vi "re_obj_LuaVIEW Task State.vi"(0 "method":T6, 1 "mode {set mode}":T2, 7 "signal":T1, 11 "script index":i32, 12 "string in":string) -> (6 "task info {get task info}":T4 {"handle mask" format="%.0b"; "allow mask" format="%.0b"; "signal flags" format="%.0b"}, 8 "set/available/pending":bool, 10 "script info":T3, 14 "string out":string, 15 "wakeup occurrence":refnum<k4>)   [LabVIEW 2012]
doc: "Instantiated per task. Holds the state of a task and allows for asynchronous communication with a task. Must be called by reference. A reference can be obtained from the task list.\n\nThis VI is only marginally part of the API: those methods that are in common use by function VIs can be deemed safe for use provided that typedefs are used so as to be forward compatible with extension of the method enum or typedef clusters (only use unbundle/bundle by name, and so on)."
uses:
  typedefs/t_LuaVIEW Task State Methods.ctl
  typedefs/t_LuaVIEW Task Modes.ctl
  typedefs/clusters/LuaVIEW Task Info.ctl
  typedefs/t_LuaVIEW Reference.ctl
  typedefs/t_LuaVIEW Task Signals.ctl
  typedefs/clusters/LuaVIEW Script Info.ctl
  typedefs/t_LuaVIEW Prepared Script Infos Methods.ctl
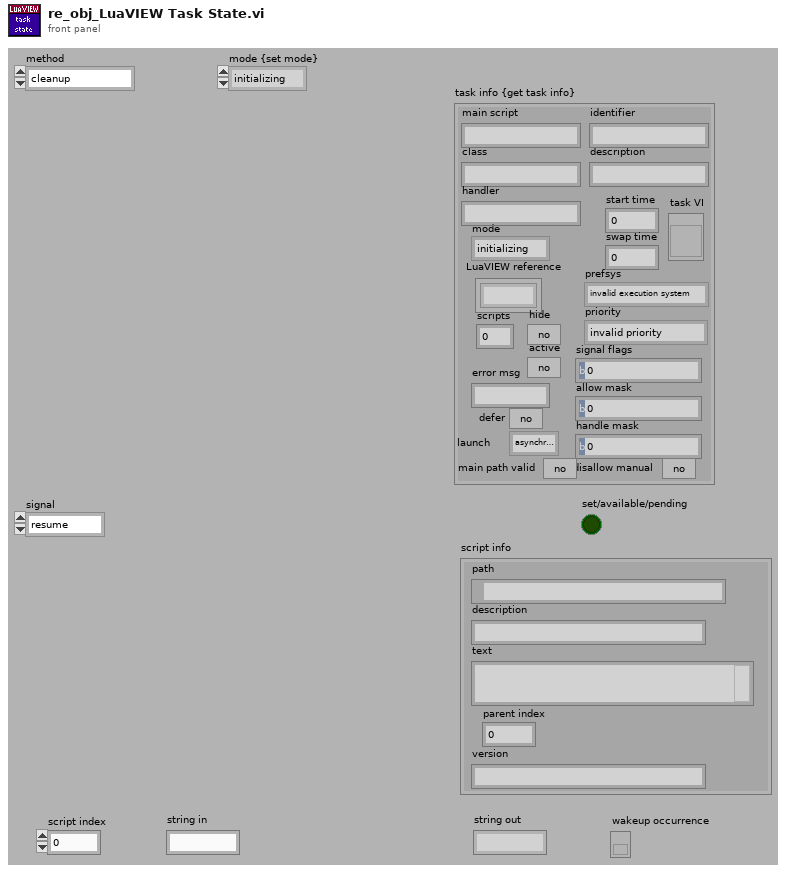
[diagram p1: front panel]
types:
  T1 = typedef "t_LuaVIEW Task Signals.ctl" = enum32{"resume", "pause", "swap", "stop", "confirm"}
  T2 = typedef "t_LuaVIEW Task Modes.ctl" = enum16{"initializing", "running", "executing", "paused", "error", "swapping"}
  T3 = typedef "LuaVIEW Script Info.ctl" = cluster{"path":path, "description":string, "text":string, "parent index":i32, "version":string}
  T4 = typedef "LuaVIEW Task Info.ctl" = cluster{"main script":string, "identifier":string, "class":string, "description":string, "mode":T2, "handler":string, "LuaVIEW reference":T5, "scripts":i32, "hide":bool, "active":bool, "error msg":string, "defer":bool, "launch":enum16{"asynchronous", "manual", "synchronous"}, "main path valid":bool, "start time":dbl, "swap time":dbl, "task VI":refnum<vi>, "prefsys":enum32{"invalid execution system", "user interface", "standard", "instrument i/o", "data acquisition", "other 1", "other 2", "same as caller"}, "priority":enum32{"invalid priority", "background priority", "normal priority", "above normal priority", "high priority", "time critical priority", "subroutine"}, "signal flags":u32, "allow mask":u32, "handle mask":u32, "disallow manual":bool}
  T5 = typedef "t_LuaVIEW Reference.ctl" = refnum<k1>
  T6 = typedef "t_LuaVIEW Task State Methods.ctl" = enum16{"cleanup", "set initial", "set mode", "set active mode", "set error", "get task info", "get script info", "set signal", "clear signal", "test handled", "test delegated", "test signal", "handle signal", "delegate signal", "allow signal", "disallow signal", "disallow all", "signals?", "delegated signals?", "protection++", "protection--", "protection=0", "message", "next message", "pop message", "message available?", "force stop", "set swap preps", "apply swap preps"}
  T7 = typedef "t_LuaVIEW Prepared Script Infos Methods.ctl" = enum16{"isempty?", "empty", "set", "discard"}
  T8 = enum32{"invalid execution system", "user interface", "standard", "instrument i/o", "data acquisition", "other 1", "other 2", "same as caller"}
  T9 = enum32{"invalid priority", "background priority", "normal priority", "above normal priority", "high priority", "time critical priority", "subroutine"}
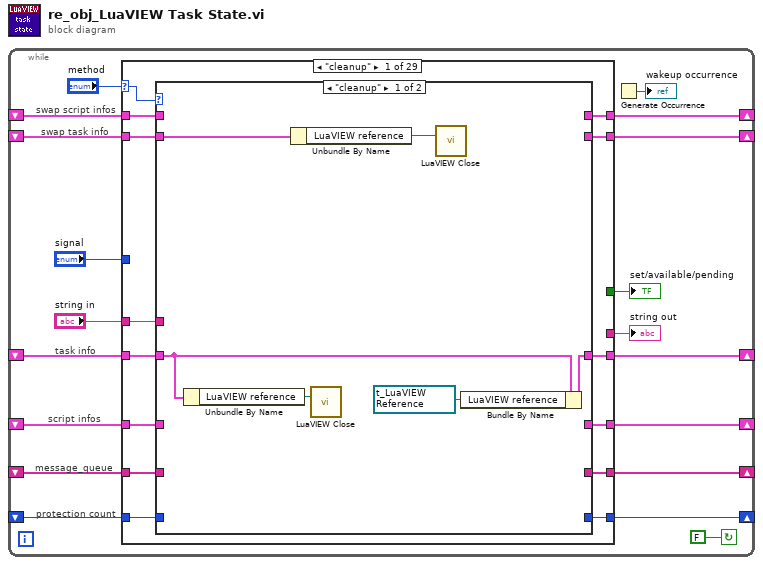
[diagram p0: block diagram]
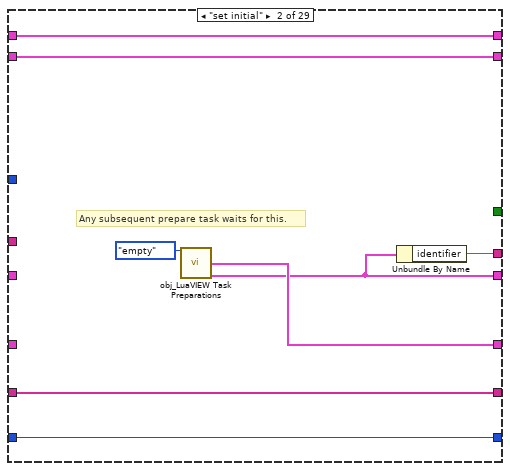
[diagram p3: hidden frame]
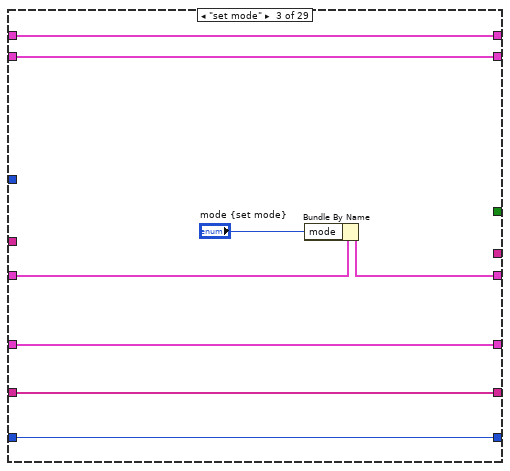
[diagram p4: hidden frame]
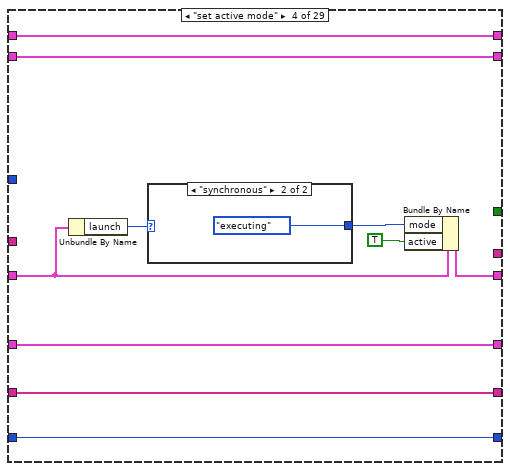
[diagram p5: hidden frame]
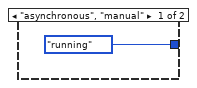
[diagram p6: hidden frame]
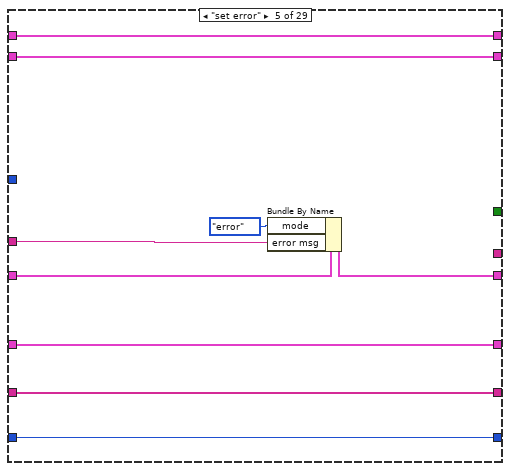
[diagram p7: hidden frame]
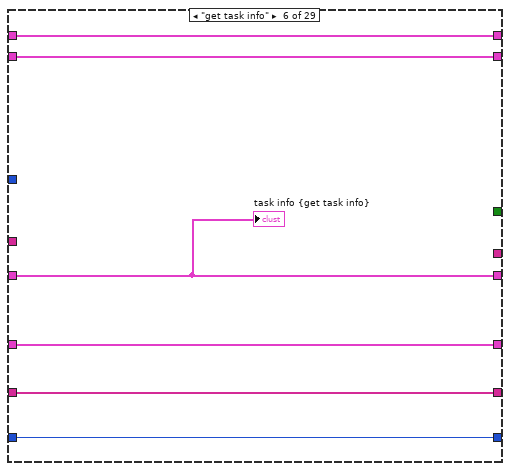
[diagram p8: hidden frame]
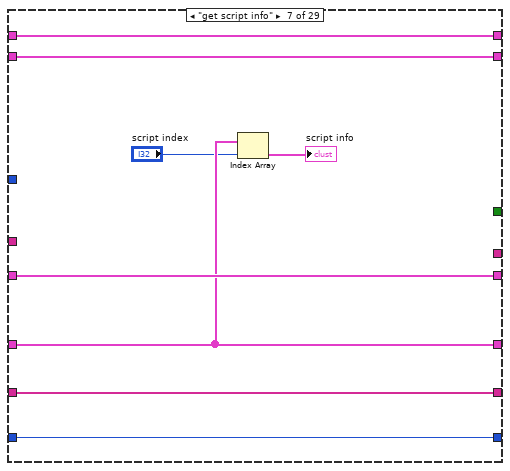
[diagram p9: hidden frame]
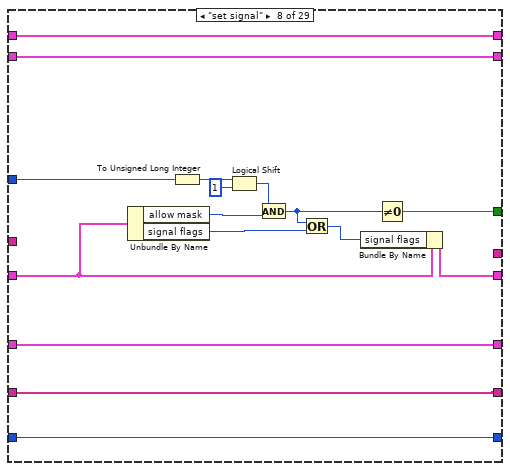
[diagram p10: hidden frame]
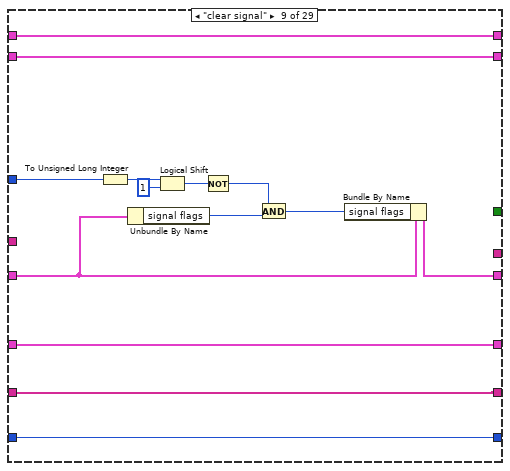
[diagram p11: hidden frame]
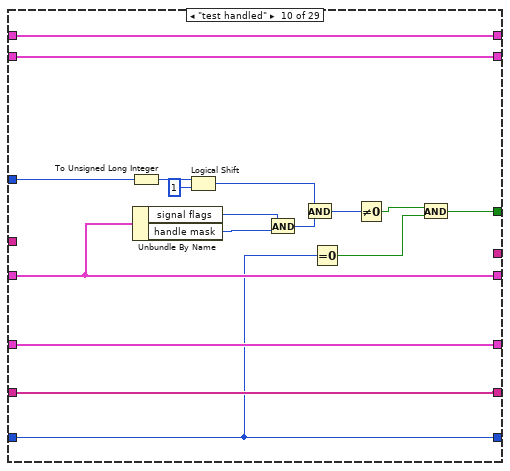
[diagram p12: hidden frame]
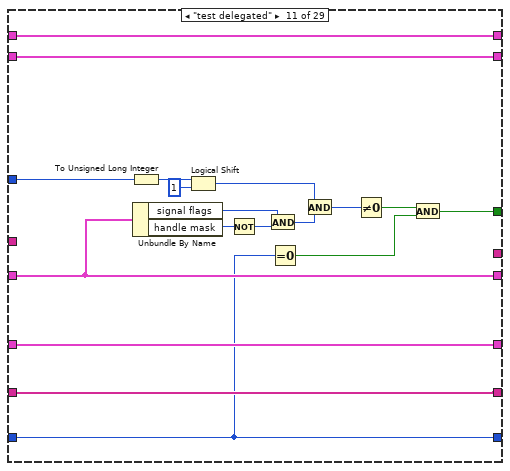
[diagram p13: hidden frame]
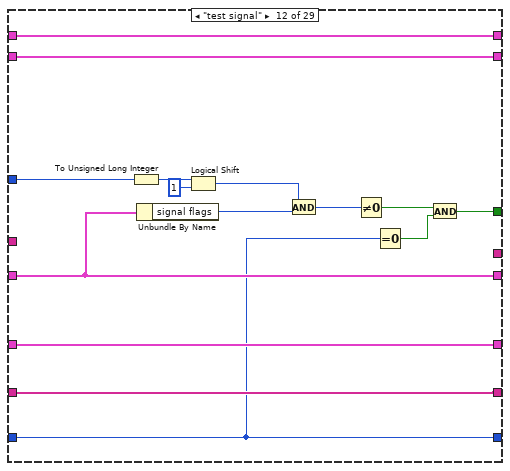
[diagram p14: hidden frame]
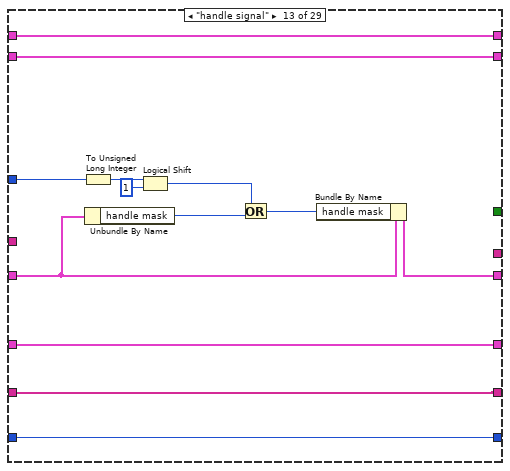
[diagram p15: hidden frame]
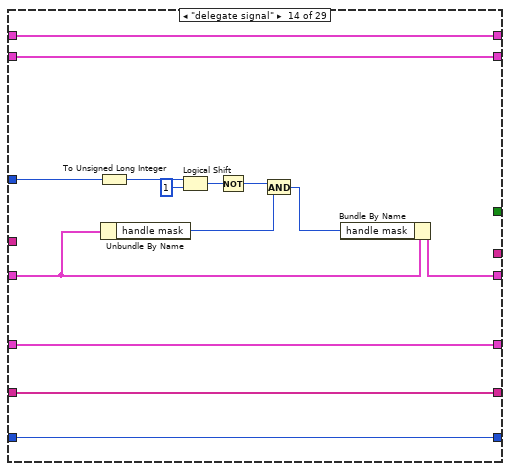
[diagram p16: hidden frame]
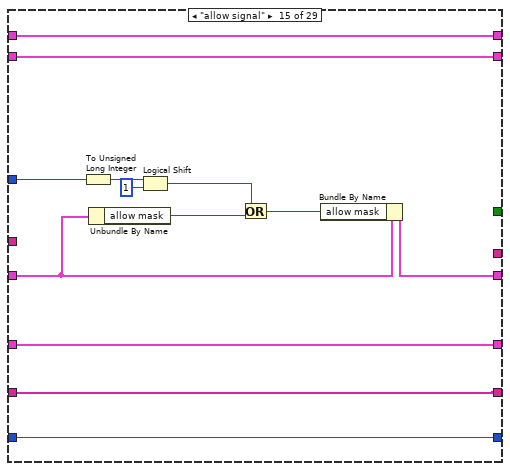
[diagram p17: hidden frame]
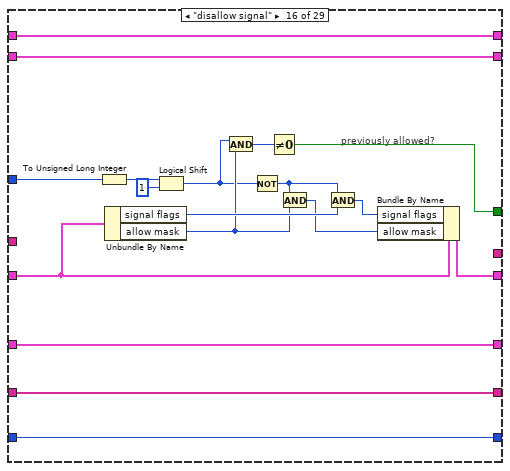
[diagram p18: hidden frame]
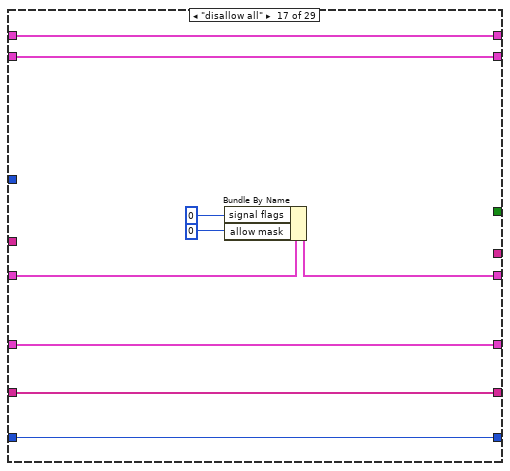
[diagram p19: hidden frame]
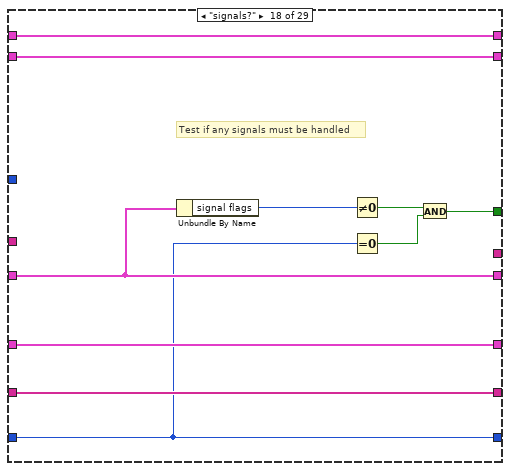
[diagram p20: hidden frame]
diagram:
  n1 = while {
    shift-right: [w17] -> _
    shift-left: _ -> [w16]
    shift-right: [w14] -> _
    shift-left: _ -> [w15]
    shift-right: [w9] -> _
    shift-left: _ -> [w10]
    shift-right: [w5] -> _
    shift-left: _ -> [w6]
    shift-right: [w1] -> _
    shift-left: _ -> [w4]
    shift-right: [w2] -> _
    shift-left: _ -> [w3]
    stop <- FALSE continue-if-true
    # "swap task info"
    # "swap script infos"
    # "protection count"
    # "message_queue"
    # "script infos"
    # "task info"
    n2 = case shown="\"cleanup\"" "method" {
      selector: "method" -> [w20 _ _ _ _ _ _ _ _ _ _ _ _ _ _ _ _ _ _ _ _ _ _ _ _ _ _ _ _]
      tunnel: [w31 w48 w59 w70 w82 w88 w96 w107 w121 w137 w155 w170 w182 w198 w209 w229 w241 w251 w264 w274 w284 w290 w298 w316 w334 w350 w364 w373 w412] -> w17
      tunnel: w16 -> [w33 _ w60 w67 w80 w88 w96 w108 w122 w137 w155 w170 w183 w199 w210 w230 w242 w251 w264 w274 w284 w290 w298 w316 w334 w350 w365 w374 w407]
      tunnel: w15 -> [w32 _ w61 w71 w81 w87 w95 w112 w126 w143 w161 w176 w189 w203 w216 w234 w243 w253 w266 w275 w285 w291 w302 w317 w335 w351 w368 w391 w413]
      tunnel: [w30 w50 w61 w71 w81 w87 w95 w112 w126 w143 w161 w176 w189 w203 w216 w234 w243 w253 w266 w275 w285 w291 w302 w317 w335 w351 w368 w391 w411] -> w14
      tunnel: "signal" -> [_ _ _ _ _ _ _ w109 w123 w138 w156 w171 w186 w200 w213 w231 _ _ _ _ _ _ _ _ _ _ _ _ _]
      tunnel: [_ _ _ _ _ _ _ w104 _ w132 w149 w167 _ _ _ w223 _ w249 w258 w270 w278 _ w295 w310 w328 w348 TRUE w376 w408] -> w12
      tunnel: w10 -> [w29 w53 w57 w69 w78 w86 w93 w100 w118 w136 w154 w168 w180 w195 w207 w222 w238 w250 w263 w273 w283 w289 w301 w313 w331 w347 w361 w384 w418]
      tunnel: [w28 w53 w57 w69 w78 w86 w93 w100 w118 w136 w154 w168 w180 w195 w207 w222 w238 w250 w263 w273 w283 w289 w300 w315 w333 w347 w361 w384 w418] -> w9
      tunnel: [_ w49 _ _ _ _ _ _ _ _ _ _ _ _ _ _ _ _ _ _ _ _ _ w314 w332 _ _ _ _] -> w8
      tunnel: "string in" -> [w27 _ _ _ w77 _ _ _ _ _ _ _ _ _ _ _ _ _ _ _ _ _ w299 _ _ _ _ _ _]
      tunnel: w6 -> [w21 w52 w56 w68 w76 w85 w92 w99 w117 w130 w147 w164 w179 w192 w206 w219 w237 w247 w256 w272 w282 _ w294 w309 w327 w346 w360 w383 _]
      tunnel: [w26 w52 w56 w68 w76 w85 w92 w99 w117 w130 w147 w164 w179 w192 w206 w219 w237 w247 w256 w271 w280 0 ("t") w294 w309 w327 w346 w360 w383 0 ("t")] -> w5
      tunnel: w4 -> [w25 w47 w55 w64 w75 w84 w91 w98 w114 w128 w145 w163 w178 w191 w205 w218 w236 w246 w255 w268 w277 w287 w293 w308 w326 w345 w353 w378 w410]
      tunnel: w3 -> [w24 w46 w54 w63 w74 w83 w90 w97 w113 w127 w144 w162 w177 w190 w204 w217 w235 w245 w254 w267 w276 w286 w292 w307 w325 w344 w352 w377 w417]
      tunnel: [w22 w46 w54 w63 w74 w83 w90 w97 w113 w127 w144 w162 w177 w190 w204 w217 w235 w245 w254 w267 w276 w286 w292 w307 w325 w344 w352 w380 w415] -> w2
      tunnel: [w23 w47 w55 w64 w75 w84 w91 w98 w114 w128 w145 w163 w178 w191 w205 w218 w236 w246 w255 w268 w277 w287 w293 w308 w326 w345 w353 w381 w416] -> w1
      frame "cleanup" {
        n3 = case shown="\"cleanup\"" w20 {
          tunnel: w33 -> [w37 w43]
          tunnel: w32 -> [_ w42]
          tunnel: [w36 w43] -> w31
          tunnel: [_ w42] -> w30
          tunnel: w29 -> [_ w41]
          tunnel: [_ w41] -> w28
          tunnel: w27 -> [_ _]
          tunnel: [_ w40] -> w26
          tunnel: w25 -> [_ w45]
          tunnel: w24 -> [w35 w44]
          tunnel: [_ w45] -> w23
          tunnel: [_ w44] -> w22
          tunnel: w21 -> [_ w40]
          frame "cleanup" {
            w34 = T5 refnum items=["LuaVIEW"] ("LuaVIEW reference")
            n4 = Unbundle By Name(w37) -> ("LuaVIEW reference"=w39:T5)
            n5 = Unbundle By Name(w35) -> ("LuaVIEW reference"=w38:T5)
            n6 = call "LuaVIEW Close.vi"("LuaVIEW reference"=w39) -> ()  [unwired: 14 in, 1 out]
            n7 = call "LuaVIEW Close.vi"("LuaVIEW reference"=w38) -> ()  [unwired: 14 in, 1 out]
            n8 = Bundle By Name(cluster=w37, "LuaVIEW reference"=w34) -> (w36:T4)
          }
          frame Default {
          }
        }
      }
      frame "set initial" {
        # "Any subsequent prepare task waits for this."
        n9 = call "obj_LuaVIEW Task Preparations.vi"("method"=t_LuaVIEW_Prepared_Script_Infos_Methods."empty") -> ("script infos out"=w50:T3[], "task info out"=w48:T4)  [unwired: 12 in, 1 out]
        n10 = Unbundle By Name(w48) -> ("identifier"=w49:string)
      }
      frame "set mode" {
        n11 = Bundle By Name(cluster=w60, "mode"="mode {set mode}") -> (w59:T4)
      }
      frame "set active mode" {
        n12 = Unbundle By Name(w67) -> ("launch"=w66:enum16{"asynchronous", "manual", "synchronous"})
        n13 = case shown="\"synchronous\"" w66 {
          tunnel: [t_LuaVIEW_Task_Modes."running" ("mode") t_LuaVIEW_Task_Modes."executing" ("mode")] -> w65
          frame "asynchronous", "manual" {
          }
          frame "synchronous" {
          }
        }
        n14 = Bundle By Name(cluster=w67, "mode"=w65, "active"=TRUE) -> (w70:T4)
      }
      frame "set error" {
        n15 = Bundle By Name(cluster=w80, "mode"=t_LuaVIEW_Task_Modes."error", "error msg"=w77) -> (w82:T4)
      }
      frame "get task info" {
        "task info {get task info}" <- w88
      }
      frame "get script info" {
        n16 = Index Array(array=w95, index="script index") -> (element=→"script info":T3)
      }
      frame "set signal" {
        n17 = Unbundle By Name(w108) -> ("allow mask"=w105:u32, "signal flags"=w103:u32)
        n18 = To Unsigned Long Integer(number=w109) -> (unsigned 32bit integer=w110:u32)
        n19 = Logical Shift(y=w110, x=u32 1) -> (x << y=w106:u32)
        n20 = And(x=w106, y=w105) -> (x .and. y?=w102:u32)
        n21 = Or(x=w102, y=w103) -> (x .or. y?=w101:u32)
        n22 = Bundle By Name(cluster=w108, "signal flags"=w101) -> (w107:T4)
        n23 = Not Equal To 0?(x=w102) -> (x != 0?=w104:bool)
      }
      frame "clear signal" {
        n24 = To Unsigned Long Integer(number=w123) -> (unsigned 32bit integer=w124:u32)
        n25 = Unbundle By Name(w122) -> ("signal flags"=w119:u32)
        n26 = Logical Shift(y=w124, x=u32 1) -> (x << y=w120:u32)
        n27 = Not(x=w120) -> (.not. x?=w115:u32)
        n28 = And(x=w115, y=w119) -> (x .and. y?=w116:u32)
        n29 = Bundle By Name(cluster=w122, "signal flags"=w116) -> (w121:T4)
      }
      frame "test handled" {
        n30 = To Unsigned Long Integer(number=w138) -> (unsigned 32bit integer=w141:u32)
        n31 = Unbundle By Name(w137) -> ("signal flags"=w135:u32, "handle mask"=w133:u32)
        n32 = Logical Shift(y=w141, x=u32 1) -> (x << y=w140:u32)
        n33 = And(x=w135, y=w133) -> (x .and. y?=w134:u32)
        n34 = And(x=w140, y=w134) -> (x .and. y?=w139:u32)
        n35 = Equal To 0?(x=w130) -> (x = 0?=w129:bool)
        n36 = Not Equal To 0?(x=w139) -> (x != 0?=w131:bool)
        n37 = And(x=w131, y=w129) -> (x .and. y?=w132:bool)
      }
      frame "test delegated" {
        n38 = To Unsigned Long Integer(number=w156) -> (unsigned 32bit integer=w159:u32)
        n39 = Unbundle By Name(w155) -> ("signal flags"=w153:u32, "handle mask"=w151:u32)
        n40 = Logical Shift(y=w159, x=u32 1) -> (x << y=w158:u32)
        n41 = Not(x=w151) -> (.not. x?=w150:u32)
        n42 = And(x=w153, y=w150) -> (x .and. y?=w152:u32)
        n43 = Equal To 0?(x=w147) -> (x = 0?=w146:bool)
        n44 = And(x=w158, y=w152) -> (x .and. y?=w157:u32)
        n45 = Not Equal To 0?(x=w157) -> (x != 0?=w148:bool)
        n46 = And(x=w148, y=w146) -> (x .and. y?=w149:bool)
      }
      frame "test signal" {
        n47 = To Unsigned Long Integer(number=w171) -> (unsigned 32bit integer=w174:u32)
        n48 = Unbundle By Name(w170) -> ("signal flags"=w169:u32)
        n49 = Logical Shift(y=w174, x=u32 1) -> (x << y=w173:u32)
        n50 = And(x=w173, y=w169) -> (x .and. y?=w172:u32)
        n51 = Not Equal To 0?(x=w172) -> (x != 0?=w166:bool)
        n52 = Equal To 0?(x=w164) -> (x = 0?=w165:bool)
        n53 = And(x=w166, y=w165) -> (x .and. y?=w167:bool)
      }
      frame "handle signal" {
        n54 = To Unsigned Long Integer(number=w186) -> (unsigned 32bit integer=w187:u32)
        n55 = Unbundle By Name(w183) -> ("handle mask"=w184:u32)
        n56 = Logical Shift(y=w187, x=u32 1) -> (x << y=w185:u32)
        n57 = Or(x=w185, y=w184) -> (x .or. y?=w181:u32)
        n58 = Bundle By Name(cluster=w183, "handle mask"=w181) -> (w182:T4)
      }
      frame "delegate signal" {
        n59 = To Unsigned Long Integer(number=w200) -> (unsigned 32bit integer=w201:u32)
        n60 = Unbundle By Name(w199) -> ("handle mask"=w196:u32)
        n61 = Logical Shift(y=w201, x=u32 1) -> (x << y=w193:u32)
        n62 = Not(x=w193) -> (.not. x?=w194:u32)
        n63 = And(x=w194, y=w196) -> (x .and. y?=w197:u32)
        n64 = Bundle By Name(cluster=w199, "handle mask"=w197) -> (w198:T4)
      }
      frame "allow signal" {
        n65 = To Unsigned Long Integer(number=w213) -> (unsigned 32bit integer=w214:u32)
        n66 = Unbundle By Name(w210) -> ("allow mask"=w211:u32)
        n67 = Logical Shift(y=w214, x=u32 1) -> (x << y=w212:u32)
        n68 = Or(x=w212, y=w211) -> (x .or. y?=w208:u32)
        n69 = Bundle By Name(cluster=w210, "allow mask"=w208) -> (w209:T4)
      }
      frame "disallow signal" {
        # "previously allowed?"
        n70 = To Unsigned Long Integer(number=w231) -> (unsigned 32bit integer=w232:u32)
        n71 = Unbundle By Name(w230) -> ("signal flags"=w228:u32, "allow mask"=w225:u32)
        n72 = Logical Shift(y=w232, x=u32 1) -> (x << y=w221:u32)
        n73 = And(x=w221, y=w225) -> (x .and. y?=w224:u32)
        n74 = Not(x=w221) -> (.not. x?=w220:u32)
        n75 = Not Equal To 0?(x=w224) -> (x != 0?=w223:bool)
        n76 = And(x=w220, y=w225) -> (x .and. y?=w226:u32)
        n77 = And(x=w220, y=w228) -> (x .and. y?=w227:u32)
        n78 = Bundle By Name(cluster=w230, "signal flags"=w227, "allow mask"=w226) -> (w229:T4)
      }
      frame "disallow all" {
        n79 = Bundle By Name(cluster=w242, "signal flags"=u32 0 ("request mask"), "allow mask"=u32 0 ("request mask")) -> (w241:T4)
      }
      frame "signals?" {
        # "Test if any signals must be handled"
        n80 = Unbundle By Name(w251) -> ("signal flags"=w244:u32)
        n81 = Not Equal To 0?(x=w244) -> (x != 0?=w252:bool)
        n82 = Equal To 0?(x=w247) -> (x = 0?=w248:bool)
        n83 = And(x=w252, y=w248) -> (x .and. y?=w249:bool)
      }
      frame "delegated signals?" {
        # "Test if any delegated signals must be handled: signals that\nthe task script does not handle itself."
        n84 = Unbundle By Name(w264) -> ("signal flags"=w262:u32, "handle mask"=w260:u32)
        n85 = Not(x=w260) -> (.not. x?=w259:u32)
        n86 = And(x=w262, y=w259) -> (x .and. y?=w261:u32)
        n87 = Equal To 0?(x=w256) -> (x = 0?=w257:bool)
        n88 = Not Equal To 0?(x=w261) -> (x != 0?=w265:bool)
        n89 = And(x=w265, y=w257) -> (x .and. y?=w258:bool)
      }
      frame "protection++" {
        n90 = Increment(x=w272) -> (x+1=w271:i32)
        n91 = Greater Or Equal?(x=w271, y=100) -> (x >= y?=w270:bool)
      }
      frame "protection--" {
        n92 = Decrement(x=w282) -> (x-1=w281:i32)
        n93 = Less Than 0?(x=w281) -> (x < 0?=w278:bool)
        n94 = Select(t=0, s=w278, f=w281) -> (s? t:f=w280:i32)
      }
      frame "protection=0" {
      }
      frame "message" {
        # "Add a message to the head of the queue"
        n95 = Unbundle By Name(w298) -> ("mode"=w297:T2)
        n96 = Not Equal?(x=w297, y=t_LuaVIEW_Task_Modes."error" ("mode")) -> (x != y?=w295:bool)
        n97 = case shown="True" w295 {
          tunnel: w301 -> [w303 w306]
          tunnel: [w303 w305] -> w300
          tunnel: w299 -> [_ w304]
          frame False {
          }
          frame True {
            n98 = Build Array (concatenate)(w304, w306) -> (w305:string[])
          }
        }
      }
      frame "next message" {
        # "Return and remove the oldest message (next when the queue is used in FIFO order)"
        n99 = Array Size(array=w313) -> (size(s)=w311:i32)
        n100 = Greater Than 0?(x=w311) -> (x > 0?=w312:bool)
        n101 = case shown="True" w312 {
          selector: w312 -> [w320 w321]
          tunnel: w313 -> [w319 w324]
          tunnel: [w319 w323] -> w315
          tunnel: ["" w322] -> w314
          tunnel: [w320 w321] -> w310
          frame False {
          }
          frame True {
            n102 = Delete From Array(array=w324) -> (deleted portion=w322:string, array with subset deleted=w323:string[])  [unwired: 2 in]
          }
        }
      }
      frame "pop message" {
        # "Return and remove the last received message (next when queue is used as a FILO stack)"
        n103 = Array Size(array=w331) -> (size(s)=w329:i32)
        n104 = Greater Than 0?(x=w329) -> (x > 0?=w330:bool)
        n105 = case shown="True" w330 {
          selector: w330 -> [w338 w340]
          tunnel: w331 -> [w337 w343]
          tunnel: [w337 w342] -> w333
          tunnel: ["" w341] -> w332
          tunnel: [w338 w340] -> w328
          frame False {
          }
          frame True {
            n106 = Delete From Array(array=w343, index=0) -> (deleted portion=w341:string, array with subset deleted=w342:string[])  [unwired: 1 in]
          }
        }
      }
      frame "message available?" {
        n107 = Array Size(array=w347) -> (size(s)=w349:i32)
        n108 = Greater Than 0?(x=w349) -> (x > 0?=w348:bool)
      }
      frame "force stop" {
        n109 = Unbundle By Name(w365) -> ("signal flags"=w363:u32, "handle mask"=w356:u32)
        n110 = To Unsigned Long Integer(number=t_LuaVIEW_Task_Signals."stop" ("signal")) -> (unsigned 32bit integer=w366:u32)
        n111 = Logical Shift(y=w366, x=u32 1) -> (x << y=w357:u32)
        n112 = Or(x=w357, y=w363) -> (x .or. y?=w362:u32)
        n113 = Not(x=w357) -> (.not. x?=w358:u32)
        n114 = And(x=w358, y=w356) -> (x .and. y?=w355:u32)
        n115 = Bundle By Name(cluster=w365, "signal flags"=w362, "handle mask"=w355) -> (w364:T4)
      }
      frame "set swap preps" {
        n116 = Unbundle By Name(w374) -> ("allow mask"=w387:u32, "signal flags"=w386:u32, "mode"=w371:T2)
        n117 = To Unsigned Long Integer(number=t_LuaVIEW_Task_Signals."swap" ("signal")) -> (unsigned 32bit integer=w389:u32)
        n118 = Logical Shift(y=w389, x=u32 1) -> (x << y=w388:u32)
        n119 = And(x=w388, y=w387) -> (x .and. y?=w385:u32)
        n120 = Or(x=w385, y=w386) -> (x .or. y?=w375:u32)
        n121 = Not Equal To 0?(x=w385) -> (x != 0?=w379:bool)
        n122 = Not Equal?(x=w371, y=t_LuaVIEW_Task_Modes."error" ("mode")) -> (x != y?=w369:bool)
        n123 = And(x=w379, y=w369) -> (x .and. y?=w372:bool)
        n124 = case shown="True" w372 {
          selector: w372 -> [w393 w400]
          tunnel: [w394 w404] -> w381
          tunnel: [w395 w403] -> w380
          tunnel: w378 -> [w394 _]
          tunnel: w377 -> [w395 w402]
          tunnel: [w393 w400] -> w376
          tunnel: w375 -> [_ w399]
          tunnel: w374 -> [w392 w398]
          tunnel: [w392 w397] -> w373
          frame False {
          }
          frame True {
            n125 = Unbundle By Name(w402) -> ("LuaVIEW reference"=w401:T5)
            n126 = Bundle By Name(cluster=w398, "signal flags"=w399, "mode"=t_LuaVIEW_Task_Modes."swapping") -> (w397:T4)
            n127 = call "obj_LuaVIEW Task Preparations.vi"("method"=t_LuaVIEW_Prepared_Script_Infos_Methods."empty") -> ("script infos out"=w404:T3[], "task info out"=w403:T4)  [unwired: 12 in, 1 out]
            n128 = call "LuaVIEW Close.vi"("LuaVIEW reference"=w401) -> ()  [unwired: 14 in, 1 out]
          }
        }
      }
      frame "apply swap preps" {
        n129 = Array Size(array=w410) -> (size(s)=w409:i32)
        n130 = Not Equal To 0?(x=w409) -> (x != 0?=w406:bool)
        n131 = case shown="True" w406 {
          selector: w406 -> [w419 w425]
          tunnel: w410 -> [w423 w437]
          tunnel: w417 -> [w422 w434]
          tunnel: [w423 _] -> w416
          tunnel: [w422 _] -> w415
          tunnel: w413 -> [w420 _]
          tunnel: w407 -> [w421 w436]
          tunnel: [w421 w429] -> w412
          tunnel: [w420 w437] -> w411
          tunnel: [w419 w425] -> w408
          frame False {
          }
          frame True {
            n132 = Unbundle By Name(w436) -> ("identifier"=w428:string, "task VI"=w433:refnum<vi>, "launch"=w432:enum16{"asynchronous", "manual", "synchronous"}, "start time"=w427:dbl, "prefsys"=w431:T8, "priority"=w430:T9, "LuaVIEW reference"=w435:T5)
            n133 = call "LuaVIEW Close.vi"("LuaVIEW reference"=w435) -> ()  [unwired: 14 in, 1 out]
            n134 = call "Library Time.vi"() -> ("time"=w426:dbl)  [unwired: 1 in]
            n135 = Bundle By Name(cluster=w434, "active"=TRUE, "identifier"=w428, "task VI"=w433, "launch"=w432, "start time"=w427, "prefsys"=w431, "priority"=w430, "swap time"=w426) -> (w429:T4)
          }
        }
      }
    }
    "set/available/pending" <- w12
    "string out" <- w8
    n136 = Generate Occurrence() -> (→"wakeup occurrence":refnum<k4>)
  }
